vi "Report Messages.vi"(8 "error in (no error)":errorcluster, 11 "Logs":T2[](array[typedef])) -> (0 "error out":errorcluster, 3 "Error/Warning ?":bool)   [LabVIEW 2013]
uses:
  control/Log.ctl
  control/Error Warning Code.ctl
panel:
  out "Error Warning Code":T1
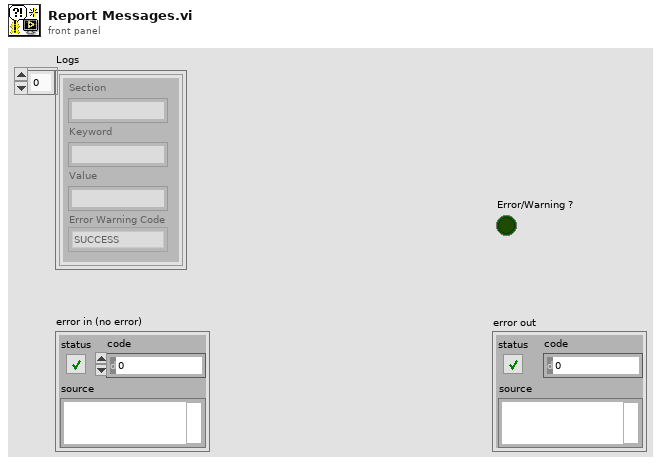
[diagram p1: front panel]
types:
  T1 = typedef "Error Warning Code.ctl" = enum16{"SUCCESS", "The data type of OD sub-entry doesn't support the compound and extended type.", "The obect type of the OD sub-entry only supports VAR.", "The multiple data object type can't be changed to single data during the editting mode.", "This OD main-entry can't belong to Manufacture.", "The main-OD or sub-OD had been created.", "The sub-OD doesn't have the main-OD.", "Make suer the object type of main-OD is multiple data.", "It cann't be saved, because of  the value of index is invalid.", "The index is not in our suppprted range.", "Filter the main-OD that address is not in our supported range.", "Don't support object types included NULL and DOMAIN.", "Don't support the Data Types included Boolean, UNICODE_STRING , DOMAIN and reserved.", "The default value can't be parsed. our of range, invalid character", "The sub-index 00 is required.", "Access Type does not support rww and rwr.", "Remove the sub OD that does not have main OD."}
  T2 = typedef "Log.ctl" = cluster{"Section":string, "Keyword":string, "Value":string, "Error Warning Code":T1}
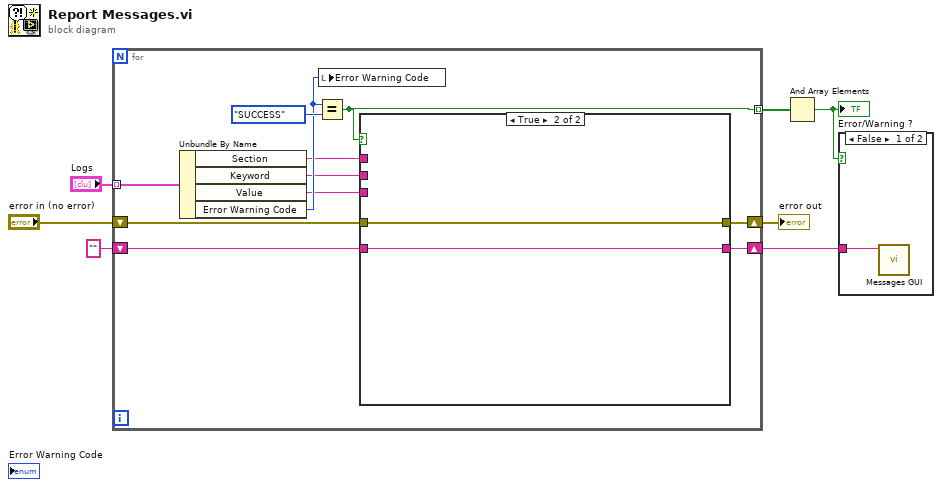
[diagram p0: block diagram]
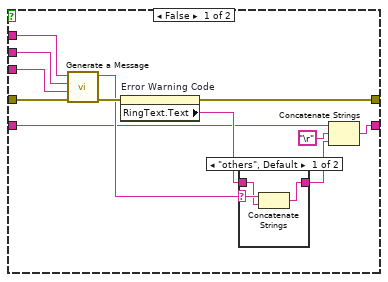
[diagram p3: hidden frame]
diagram:
  n1 = for {
    tunnel: "Logs" -> [w18] mode=indexing
    shift-right: [w10] -> w5
    shift-left: "error in (no error)" -> [w15]
    shift-right: [w8] -> w1
    shift-left: "" -> [w9]
    tunnel: [w16] -> w3 mode=indexing
    n2 = Unbundle By Name(w18) -> ("Section"=w13:string, "Keyword"=w12:string, "Value"=w11:string, "Error Warning Code"=w14:T1)
    n3 = Equal?(x=w14, y=Error_Warning_Code."SUCCESS" ("Error Warning Code")) -> (x = y?=w16:bool)
    n4 = local write "Error Warning Code"(w14) -> ()
    n5 = case shown="True" w16 {
      tunnel: w15 -> [w26 w36]
      tunnel: [w30 w36] -> w10
      tunnel: w13 -> [w29 _]
      tunnel: w12 -> [w28 _]
      tunnel: w11 -> [w27 _]
      tunnel: [w19 w35] -> w8
      tunnel: w9 -> [w22 w35]
      frame False {
        n6 = call "Generate a Message.vi"("error in (no error)"=w26, "Value"=w27, "Keyword"=w28, "Section"=w29) -> ("error out"=w25:errorcluster, "Message"=w24:string)  [unwired: 6 in]
        n7 = property on="Error Warning Code" class="Enum (strict)"(error in=w25) -> (error out=w30:errorcluster, "RingText.Text"=w23:string)  [unwired: 1 in, 1 out]
        n8 = case shown="\"others\", Default" w24 {
          selector: w24 -> [w32 _]
          tunnel: [w33 w34] -> w20
          tunnel: w23 -> [w31 w34]
          frame "others", Default {
            n9 = Concatenate Strings(w32, w31) -> (w33:string)
          }
          frame "" {
          }
        }
        n10 = Concatenate Strings(w22, "\r", w20) -> (w19:string)
      }
      frame True {
      }
    }
  }
  "error out" <- w5
  n11 = And Array Elements(Boolean array=w3) -> (logical AND=w2:bool)
  "Error/Warning ?" <- w2
  n12 = case shown="False" w2 {
    tunnel: w1 -> [w37 _]
    frame False {
      n13 = call "Messages GUI.vi"("Messages"=w37) -> ()  [unwired: 11 in]
    }
    frame True {
    }
  }
